vi "LAN Trigger Connected.vi"(8 "error in":errorcluster, 9 "Trigger # (1)":u32=1 min=1 max=8, 10 "Node In":string, 11 "VISA resource name":refnum<visa-resource-name>) -> (0 "error out":errorcluster, 1 "Connected":bool, 2 "Node Out":string, 3 "VISA resource name out":refnum<visa-resource-name>, 4 "Command String":string)   [LabVIEW 2009, in "Keithley 2600 Series.lvlib"]
doc: "The VI checks the connection status of a LAN trigger.\n\n<b>Functions and Attributes Used</b>\nlan.trigger[n].connected"
uses:
  <instrlib>/Keithley 2600 Series/Keithley 2600 Series.lvlib
  <instrlib>/Keithley 2600 Series/Private/GlobalVariables.vi
panel:
  # "(c) 2008 Keithley Instruments, Inc.  ALL RIGHTS RESERVED."
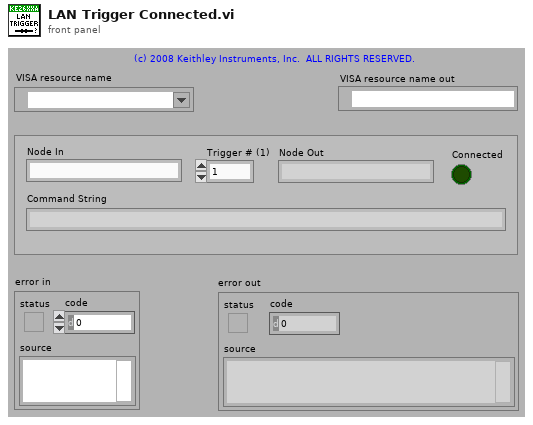
[diagram p1: front panel]
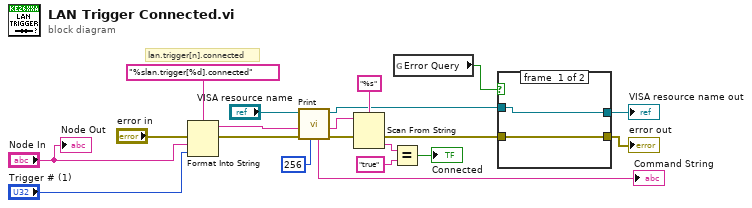
[diagram p0: block diagram]
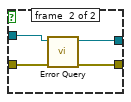
[diagram p2: hidden frame]
diagram:
  # "lan.trigger[n].connected"
  n1 = Format Into String(format string="%slan.trigger[%d].connected", error in="error in", "Node In", "Trigger # (1)") -> (resulting string=w8:string, error out=w7:errorcluster)  [unwired: 1 in]
  n2 = call <instrlib>:"Print.vi"("Byte Count (1024)"=u32 256, "error in (no error)"=w7, "Input"=w8, "VISA resource name"="VISA resource name") -> ("error out"=w3:errorcluster, "Output"=w4:string, "VISA resource name out"=w1:refnum<visa-resource-name>, "Command String"=→"Command String":string)  [unwired: 1 in, 3 out]
  n3 = Scan From String(format string="%s", input string=w4, error in=w3) -> (error out=w12:errorcluster, output 1=w15:string)  [unwired: 1 in, 3 out]
  n4 = Equal?(x=w15, y="true") -> (x = y?=→"Connected":bool)
  n5 = global read "GlobalVariables.vi" "Error Query"() -> (w11:bool)
  n6 = case shown="True" w11 {
    tunnel: w12 -> [w22 w26]
    tunnel: [w21 w25] -> w10
    tunnel: [w22 w24] -> w9
    tunnel: w1 -> [w21 w23]
    frame #0 {
    }
    frame #1 {
      n7 = call <instrlib>:"Error Query.vi"("error in (no error)"=w26, "VISA resource name"=w23) -> ("error out"=w24:errorcluster, "VISA resource name out"=w25:refnum<visa-resource-name>)  [unwired: 8 out]
    }
  }
  "VISA resource name out" <- w10
  "error out" <- w9
  "Node Out" <- "Node In"
